vi "Do Core.vi"(8 "error in (no error)":errorcluster, 10 "Actor in":refnum<class "Actor.lvclass">, 11 "Message":refnum<class "Pre Iteration Msg.lvclass">) -> (0 "error out":errorcluster, 2 "Actor out":refnum<class "Actor.lvclass">, 3 "Iterate":bool)   [LabVIEW 2023, in "Example Iterator NR Actor Implicit Iteration.lvlib" / "Pre Iteration Msg.lvclass"]
doc: "(<B>Filename</B>: Actor Framework.lvlib:Reply Msg.lvclass:Do Core.vi)\n\nDefines what an actor does when it receives <B>Reply Message</B>. This method also defines the <B>Reply</B> that is returned to the actor that sent <B>Reply Message</B>.\n\nBy default, this method does nothing, and <B>Reply</B> is the ancestor Message class. A child class must override this method to define behavior and specify a child of the Message class to return in the <B>Reply</B> output."
uses:
  Pre Iteration Msg.lvclass
  <vilib>/ActorFramework/Actor/Actor.lvclass
  Example Actor/Example Actor.lvclass
  C:/Program Files/National Instruments/LabVIEW 2023/vi.lib/ActorFramework/Actor/Actor.lvclass
  Pre Iteration Msg.lvclass/Pre Iteration Msg.ctl
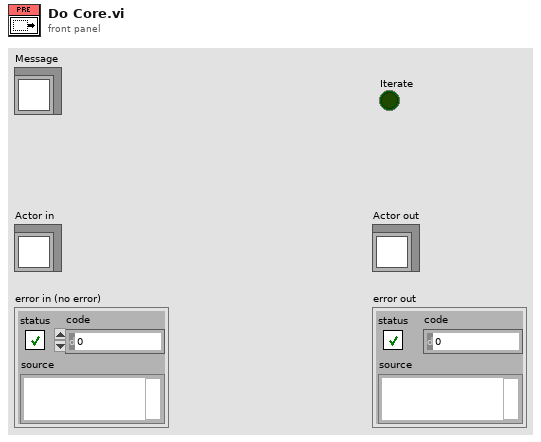
[diagram p1: front panel]
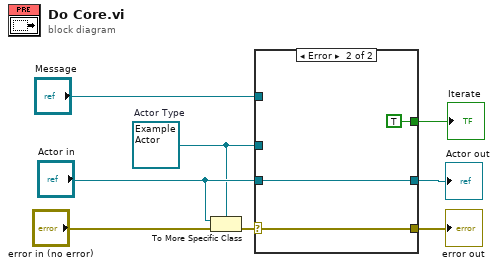
[diagram p0: block diagram]
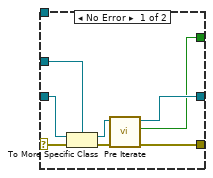
[diagram p2: hidden frame]
diagram:
  w5 = refnum<class "Example Actor.lvclass"> refnum  # Actor Type
  n1 = To More Specific Class(target class=w5, reference="Actor in", error in="error in (no error)") -> (error out=w7:errorcluster)  [unwired: 1 out]
  n2 = case shown="Error" w7 {
    selector: w7 -> [w16 w19]
    tunnel: [w11 w19] -> w2
    tunnel: [w10 w18] -> w3
    tunnel: "Actor in" -> [w15 w18]
    tunnel: w5 -> [w14 _]
    tunnel: "Message" -> [_ _]
    tunnel: [w9 TRUE ("Ready for iterations")] -> w1
    frame No Error {
      n3 = To More Specific Class ("Actor Cast")(target class=w14, reference=w15, error in=w16) -> (specific class reference=w13:refnum<class "Example Actor.lvclass">, error out=w12:errorcluster)
      n4 = call "Pre Iterate.vi"("error in (no error)"=w12, "Example Actor in"=w13) -> ("error out"=w11:errorcluster, "Ready for iterations"=w9:bool, "Example Actor out"=w10:refnum<class "Example Actor.lvclass">)  [unwired: 7 in]
    }
    frame Error {
    }
  }
  "error out" <- w2
  "Actor out" <- w3
  "Iterate" <- w1
